vi "RL Front Panel.vi"() -> ()   [LabVIEW 2023]
panel:
  in  "stop":bool
  in  "start":bool
  in  "Sample Mode":string(combo)
  in  "Num Sensors":dbl
  in  "16":bool
  in  "15":bool
  in  "14":bool
  in  "13":bool
  in  "12":bool
  in  "11":bool
  in  "10":bool
  in  "9":bool
  in  "8":bool
  in  "7":bool
  in  "6":bool
  in  "5":bool
  in  "4":bool
  in  "3":bool
  in  "2":bool
  in  "1":bool
  in  "config":bool
  in  "setAllSamp":bool
  in  "setSamp":bool
  in  "selectAll":bool
  in  "Sensor Num":i32
  in  "selectSensor":bool
  in  "connectSensor":bool
  out "Pipeline Status":string
  in  "Connect":bool
  # "Delsys"
  # "Sensors"
  # "Data Collection"
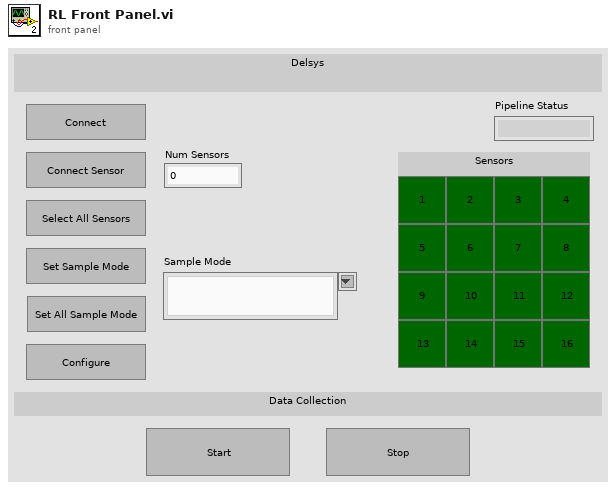
[diagram p1: front panel]
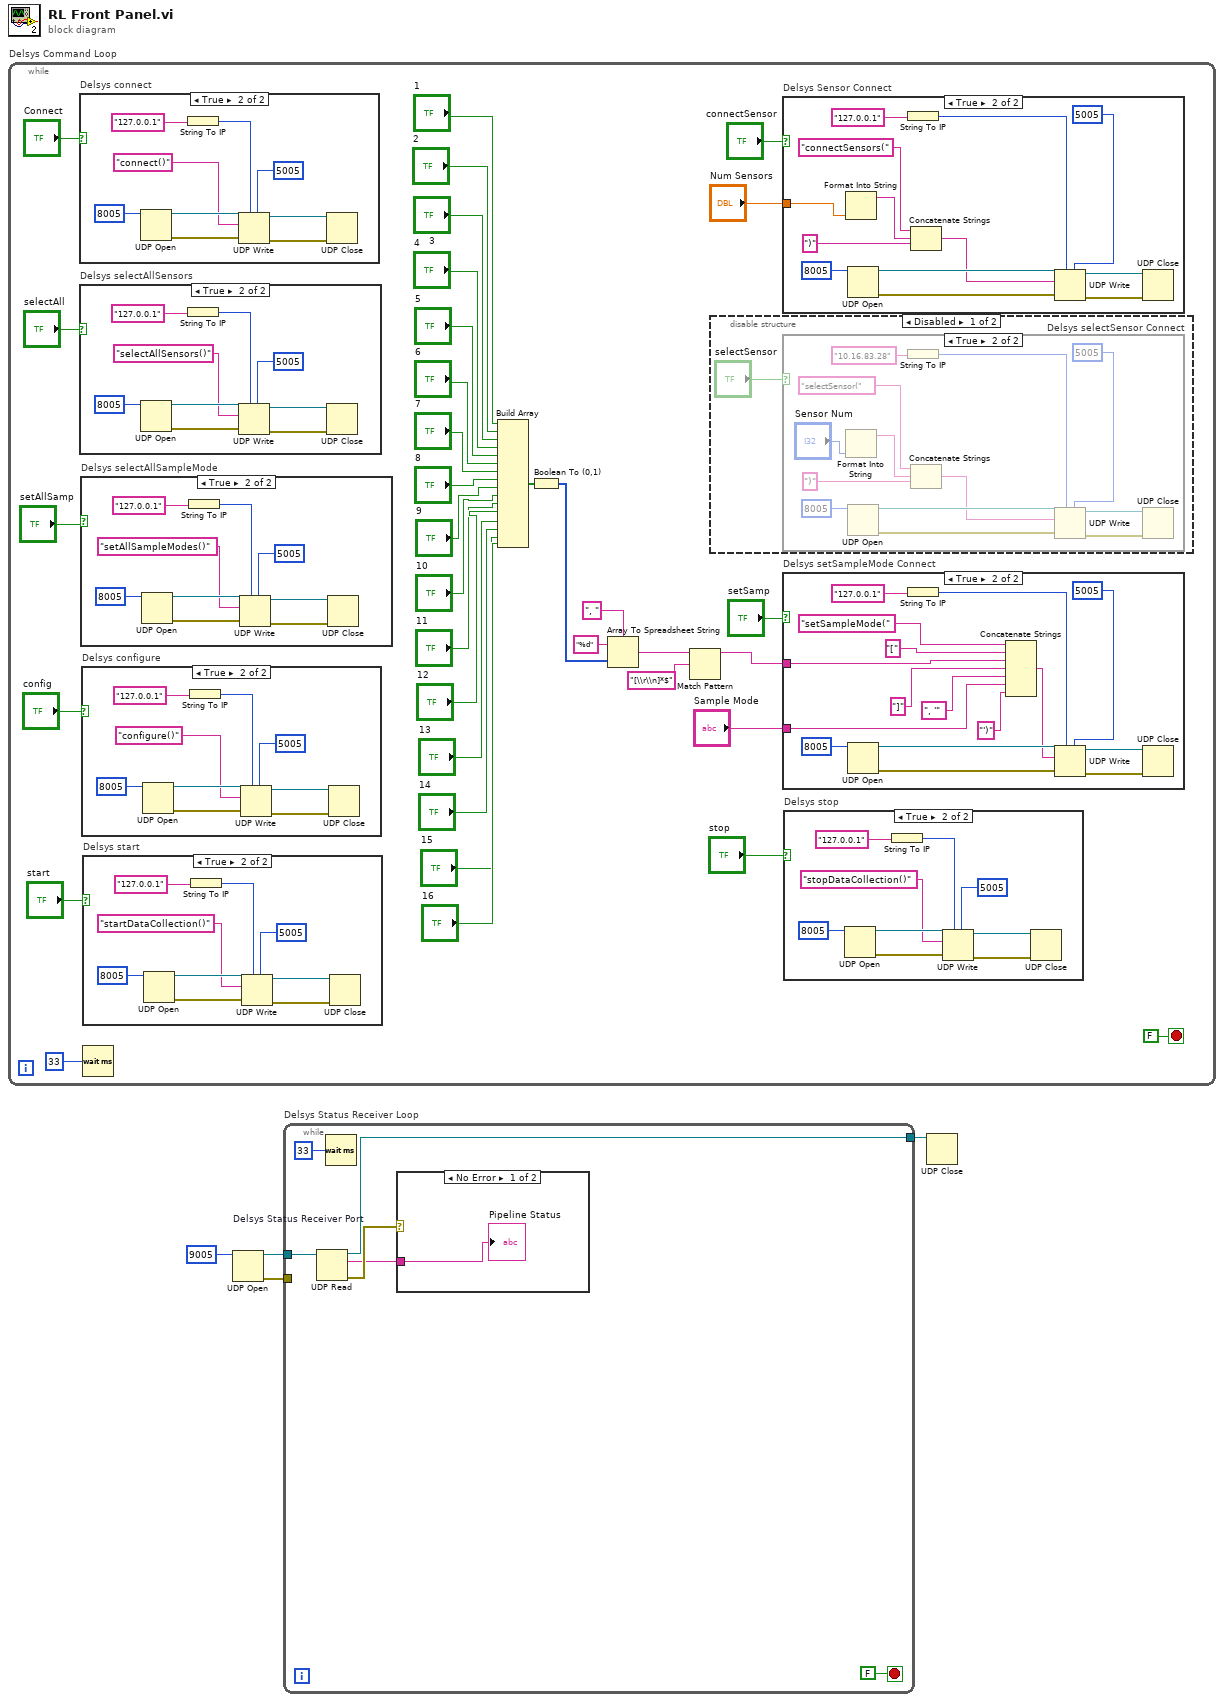
[diagram p0: block diagram]
diagram:
  n1 = while "Delsys Command Loop" {
    stop <- FALSE stop-if-true
    n2 = case "Delsys connect" shown="True" "Connect" {
      frame False {
      }
      frame True {
        n3 = UDP Open(11:8005) -> (port=w136:refnum<k16>, 0:w134:errorcluster)  [unwired: 4 in, 1 out]
        n4 = String To IP(1:"127.0.0.1") -> (0:w129:u32)
        n5 = UDP Write(address=w129, port or service name=5005, connection ID=w136, data in="connect()", 8:w134) -> (error out=w133:errorcluster, 3:w135:refnum<k16>)  [unwired: 1 in]
        n6 = UDP Close(connection ID=w135, 8:w133) -> ()  [unwired: 2 out]
      }
    }
    n7 = case "Delsys selectAllSensors" shown="True" "selectAll" {
      frame False {
      }
      frame True {
        n8 = UDP Open(11:8005) -> (port=w114:refnum<k16>, 0:w112:errorcluster)  [unwired: 4 in, 1 out]
        n9 = String To IP(1:"127.0.0.1") -> (0:w107:u32)
        n10 = UDP Write(address=w107, port or service name=5005, connection ID=w114, data in="selectAllSensors()", 8:w112) -> (error out=w111:errorcluster, 3:w113:refnum<k16>)  [unwired: 1 in]
        n11 = UDP Close(connection ID=w113, 8:w111) -> ()  [unwired: 2 out]
      }
    }
    n12 = case "Delsys selectAllSampleMode" shown="True" "setAllSamp" {
      frame False {
      }
      frame True {
        n13 = UDP Open(11:8005) -> (port=w89:refnum<k16>, 0:w87:errorcluster)  [unwired: 4 in, 1 out]
        n14 = String To IP(1:"127.0.0.1") -> (0:w82:u32)
        n15 = UDP Write(address=w82, port or service name=5005, connection ID=w89, data in="setAllSampleModes()", 8:w87) -> (error out=w86:errorcluster, 3:w88:refnum<k16>)  [unwired: 1 in]
        n16 = UDP Close(connection ID=w88, 8:w86) -> ()  [unwired: 2 out]
      }
    }
    n17 = case "Delsys configure" shown="True" "config" {
      frame False {
      }
      frame True {
        n18 = UDP Open(11:8005) -> (port=w80:refnum<k16>, 0:w78:errorcluster)  [unwired: 4 in, 1 out]
        n19 = String To IP(1:"127.0.0.1") -> (0:w73:u32)
        n20 = UDP Write(address=w73, port or service name=5005, connection ID=w80, data in="configure()", 8:w78) -> (error out=w77:errorcluster, 3:w79:refnum<k16>)  [unwired: 1 in]
        n21 = UDP Close(connection ID=w79, 8:w77) -> ()  [unwired: 2 out]
      }
    }
    n22 = case "Delsys start" shown="True" "start" {
      frame False {
      }
      frame True {
        n23 = UDP Open(11:8005) -> (port=w57:refnum<k16>, 0:w55:errorcluster)  [unwired: 4 in, 1 out]
        n24 = String To IP(1:"127.0.0.1") -> (0:w50:u32)
        n25 = UDP Write(address=w50, port or service name=5005, connection ID=w57, data in="startDataCollection()", 8:w55) -> (error out=w54:errorcluster, 3:w56:refnum<k16>)  [unwired: 1 in]
        n26 = UDP Close(connection ID=w56, 8:w54) -> ()  [unwired: 2 out]
      }
    }
    n27 = Wait (ms)(milliseconds to wait=33) -> ()  [unwired: 1 out]
    n28 = Build Array("1", "2", "3", "4", "5", "6", "7", "8", "9", "10", "11", "12", "13", "14", "15", "16") -> (w15:bool[])
    n29 = Boolean To (0,1)(Boolean=w15) -> (0, 1=w11:i16[])
    n30 = Array To Spreadsheet String(delimiter (Tab)=", ", array=w11, 3:"%d" ("format string")) -> (spreadsheet string=w7:string)
    n31 = Match Pattern(string=w7, regular expression="[\\r\\n]*$") -> (before substring=w8:string)  [unwired: 1 in, 3 out]
    n32 = disable-structure shown="Disabled" {
      frame Disabled {
        n33 = case "Delsys selectSensor Connect" shown="True" "selectSensor" {
          frame False {
          }
          frame True {
            n34 = Format Into String("Sensor Num") -> (resulting string=w62:string)  [unwired: 3 in, 1 out]
            n35 = UDP Open(11:8005) -> (port=w71:refnum<k16>, 0:w69:errorcluster)  [unwired: 4 in, 1 out]
            n36 = String To IP(1:"10.16.83.28") -> (0:w64:u32)
            n37 = Concatenate Strings("selectSensor(", w62, ")") -> (w60:string)
            n38 = UDP Write(address=w64, port or service name=5005, connection ID=w71, data in=w60, 8:w69) -> (error out=w68:errorcluster, 3:w70:refnum<k16>)  [unwired: 1 in]
            n39 = UDP Close(connection ID=w70, 8:w68) -> ()  [unwired: 2 out]
          }
        }
      }
      frame Enabled {
      }
    }
    n40 = case "Delsys Sensor Connect" shown="True" "connectSensor" {
      tunnel: "Num Sensors" -> [_ w115]
      frame False {
      }
      frame True {
        n41 = Format Into String(w115) -> (resulting string=w118:string)  [unwired: 3 in, 1 out]
        n42 = UDP Open(11:8005) -> (port=w127:refnum<k16>, 0:w125:errorcluster)  [unwired: 4 in, 1 out]
        n43 = String To IP(1:"127.0.0.1") -> (0:w120:u32)
        n44 = Concatenate Strings("connectSensors(", w118, ")") -> (w116:string)
        n45 = UDP Write(address=w120, port or service name=5005, connection ID=w127, data in=w116, 8:w125) -> (error out=w124:errorcluster, 3:w126:refnum<k16>)  [unwired: 1 in]
        n46 = UDP Close(connection ID=w126, 8:w124) -> ()  [unwired: 2 out]
      }
    }
    n47 = case "Delsys setSampleMode Connect" shown="True" "setSamp" {
      tunnel: "Sample Mode" -> [_ w96]
      tunnel: w8 -> [_ w93]
      frame False {
      }
      frame True {
        n48 = UDP Open(11:8005) -> (port=w105:refnum<k16>, 0:w103:errorcluster)  [unwired: 4 in, 1 out]
        n49 = String To IP(1:"127.0.0.1") -> (0:w98:u32)
        n50 = Concatenate Strings("setSampleMode(", "[" ("string"), w93, "]" ("string"), ", '" ("string"), w96, "')") -> (w90:string)
        n51 = UDP Write(address=w98, port or service name=5005, connection ID=w105, data in=w90, 8:w103) -> (error out=w102:errorcluster, 3:w104:refnum<k16>)  [unwired: 1 in]
        n52 = UDP Close(connection ID=w104, 8:w102) -> ()  [unwired: 2 out]
      }
    }
    n53 = case "Delsys stop" shown="True" "stop" {
      frame False {
      }
      frame True {
        n54 = UDP Open(11:8005) -> (port=w48:refnum<k16>, 0:w46:errorcluster)  [unwired: 4 in, 1 out]
        n55 = String To IP(1:"127.0.0.1") -> (0:w41:u32)
        n56 = UDP Write(address=w41, port or service name=5005, connection ID=w48, data in="stopDataCollection()", 8:w46) -> (error out=w45:errorcluster, 3:w47:refnum<k16>)  [unwired: 1 in]
        n57 = UDP Close(connection ID=w47, 8:w45) -> ()  [unwired: 2 out]
      }
    }
  }
  n58 = UDP Open "Delsys Status Receiver Port"(11:9005) -> (port=w3:refnum<k16>, 0:w1:errorcluster)  [unwired: 4 in, 1 out]
  n59 = while "Delsys Status Receiver Loop" {
    tunnel: [w142] -> w4
    tunnel: w3 -> [w141]
    tunnel: w1 -> [_]
    stop <- FALSE stop-if-true
    n60 = UDP Read(connection ID=w141) -> (data out=w138:string, error out=w139:errorcluster, 3:w142:refnum<k16>)  [unwired: 3 in, 2 out]
    n61 = Wait (ms)(milliseconds to wait=33) -> ()  [unwired: 1 out]
    n62 = case shown="No Error" w139 {
      tunnel: w138 -> [w143 _]
      frame No Error {
        "Pipeline Status" <- w143
      }
      frame Error {
      }
    }
  }
  n63 = UDP Close(connection ID=w4) -> ()  [unwired: 1 in, 2 out]
